vi "Nested Loops Solution.vi"() -> (3 "Solutions (Quantity)":i32[][](array[numeric]))   [LabVIEW 2018]
uses:
  ctl/Coin data--cluster.ctl
panel:
  out "No. solutions":i32
  out "Values (p)":i32[](array[numeric])
  out "Progress - current iteration values":i32[](array[numeric])
  out "Time taken (s)":dbl
  # "Beer money - Nested Loops/ Speedy solution"
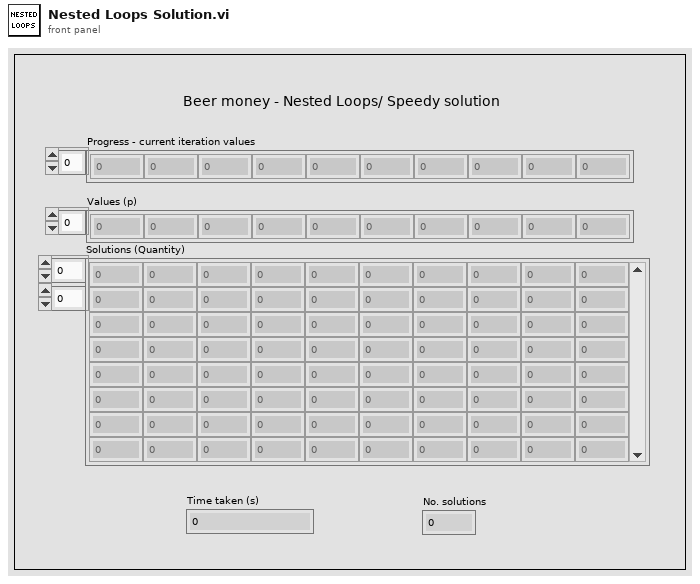
[diagram p1: front panel]
types:
  T1 = typedef "Coin data--cluster.ctl" = cluster{"Coin/note":i32, "Quantity":i32}
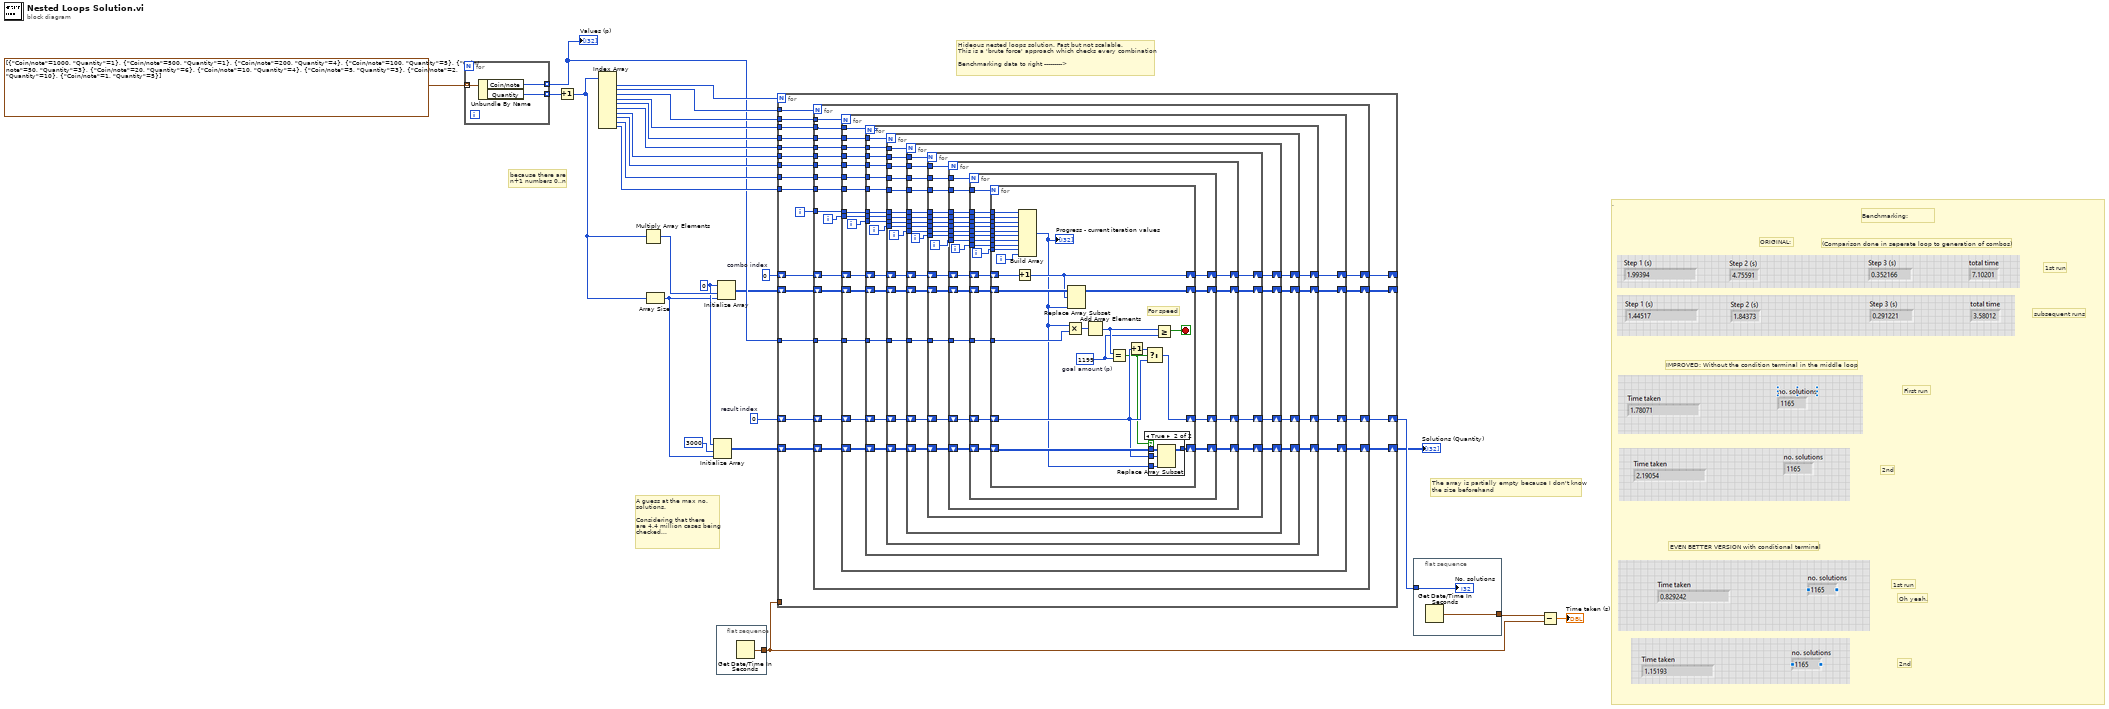
[diagram p0: block diagram]
diagram:
  w4 = 0 ("dimension size")
  w8 = 0  # result index
  w13 = 0  # combo index
  # "2nd"
  # "subsequent runs"
  # "The array is partially empty because I don't know\nthe size beforehand"
  # "Benchmarking:"
  # "(Comparison done in seperate loop to generation of combos)"
  # "1st run"
  # "Oh yeah."
  # "EVEN BETTER VERSION with conditional terminal"
  # "2nd"
  # "First run"
  # "IMPROVED: Without the condition terminal in the middle loop"
  # "A guess at the max no.\nsolutions.\n\nConsidering that there \nare 4.4 million cases being \nchecked..."
  # "ORIGINAL:"
  # "1st run"
  # "Hideous nested loops solution. Fast but not scalable.\nThis is a 'brute force' approach which checks every combination\n\nBenchmarking data to right --------->"
  # "because there are \nn+1 numbers 0..n"
  # "."
  n1 = for {
    tunnel: T1[] [{"Coin/note"=1000, "Quantity"=1}, {"Coin/note"=500, "Quantity"=1}, {"Coin/note"=200, "Quantity"=4}, {"Coin/note"=100, "Quantity"=5}, {"Coin/note"=50, "Quantity"=3}, {"Coin/note"=20, "Quantity"=6}, {"Coin/note"=10, "Quantity"=4}, {"Coin/note"=5, "Quantity"=3}, {"Coin/note"=2, "Quantity"=10}, {"Coin/note"=1, "Quantity"=5}] -> [w30] mode=indexing
    tunnel: [w29] -> w9 mode=indexing
    tunnel: [w28] -> w26 mode=indexing
    n2 = Unbundle By Name(w30) -> ("Coin/note"=w29:i32, "Quantity"=w28:i32)
  }
  "Values (p)" <- w9
  n3 = Increment(x=w26) -> (x+1=w12:i32[])
  n4 = Index Array(array=w12) -> (element #1=w24:i32, element #2=w23:i32, element #3=w22:i32, element #4=w21:i32, element #5=w20:i32, element #6=w19:i32, element #7=w18:i32, element #8=w17:i32, element #9=w16:i32, element #10=w15:i32)  [unwired: 10 in]
  n5 = Multiply Array Elements(1:w12) -> (0:w25:i32)
  n6 = Array Size(array=w12) -> (size(s)=w3:i32)
  n7 = Initialize Array(w4, 3000 ("dimension size"), w3) -> (w5:i32[][])
  n8 = flat-sequence {
    tunnel: [w31] -> w14
    frame #0 {
      n9 = Get Date/Time In Seconds() -> (seconds since 1Jan1904=w31:timestamp)
    }
  }
  n10 = Initialize Array(w4, w25, w3) -> (w7:i32[][])
  n11 = for {
    N: w24 -> [_]
    tunnel: w23 -> [w46]
    tunnel: w22 -> [w47]
    tunnel: w21 -> [w48]
    tunnel: w20 -> [w45]
    tunnel: w19 -> [w44]
    tunnel: w18 -> [w43]
    tunnel: w17 -> [w42]
    tunnel: w16 -> [w41]
    tunnel: w15 -> [w40]
    shift-right: [w50] -> _
    shift-left: w7 -> [w39]
    tunnel: w14 -> [_]
    shift-right: [w37] -> _
    shift-left: w13 -> [w38]
    tunnel: w9 -> [w36]
    shift-right: [w32] -> w6
    shift-left: w8 -> [w35]
    shift-right: [w33] -> w1
    shift-left: w5 -> [w34]
    i -> [w49]
    n12 = for {
      N: w46 -> [_]
      tunnel: w49 -> [w69]
      tunnel: w47 -> [w65]
      tunnel: w48 -> [w66]
      tunnel: w45 -> [w64]
      tunnel: w44 -> [w63]
      tunnel: w43 -> [w62]
      tunnel: w42 -> [w61]
      tunnel: w41 -> [w60]
      tunnel: w40 -> [w59]
      shift-right: [w68] -> w50
      shift-left: w39 -> [w58]
      shift-right: [w56] -> w37
      shift-left: w38 -> [w57]
      tunnel: w36 -> [w55]
      shift-right: [w51] -> w32
      shift-left: w35 -> [w54]
      shift-right: [w52] -> w33
      shift-left: w34 -> [w53]
      i -> [w67]
      n13 = for {
        N: w65 -> [_]
        tunnel: w69 -> [w88]
        tunnel: w67 -> [w87]
        tunnel: w66 -> [w84]
        tunnel: w64 -> [w83]
        tunnel: w63 -> [w82]
        tunnel: w62 -> [w81]
        tunnel: w61 -> [w80]
        tunnel: w60 -> [w79]
        tunnel: w59 -> [w78]
        shift-right: [w86] -> w68
        shift-left: w58 -> [w77]
        shift-right: [w75] -> w56
        shift-left: w57 -> [w76]
        tunnel: w55 -> [w74]
        shift-right: [w70] -> w51
        shift-left: w54 -> [w73]
        shift-right: [w71] -> w52
        shift-left: w53 -> [w72]
        i -> [w85]
        n14 = for {
          N: w84 -> [_]
          tunnel: w88 -> [w107]
          tunnel: w85 -> [w106]
          tunnel: w87 -> [w105]
          shift-right: [w104] -> w86
          shift-left: w77 -> [w103]
          tunnel: w83 -> [w102]
          tunnel: w82 -> [w101]
          tunnel: w81 -> [w100]
          tunnel: w80 -> [w99]
          tunnel: w79 -> [w98]
          tunnel: w78 -> [w97]
          shift-right: [w94] -> w75
          shift-left: w76 -> [w95]
          tunnel: w74 -> [w93]
          shift-right: [w89] -> w70
          shift-left: w73 -> [w92]
          shift-right: [w90] -> w71
          shift-left: w72 -> [w91]
          i -> [w96]
          n15 = for {
            N: w102 -> [_]
            tunnel: w107 -> [w126]
            tunnel: w106 -> [w125]
            tunnel: w105 -> [w124]
            shift-right: [w123] -> w104
            shift-left: w103 -> [w122]
            tunnel: w101 -> [w121]
            tunnel: w100 -> [w120]
            tunnel: w99 -> [w119]
            tunnel: w98 -> [w118]
            tunnel: w97 -> [w117]
            tunnel: w96 -> [w115]
            shift-right: [w113] -> w94
            shift-left: w95 -> [w114]
            tunnel: w93 -> [w112]
            shift-right: [w108] -> w89
            shift-left: w92 -> [w111]
            shift-right: [w109] -> w90
            shift-left: w91 -> [w110]
            i -> [w116]
            n16 = for {
              N: w121 -> [_]
              tunnel: w126 -> [w145]
              tunnel: w125 -> [w144]
              tunnel: w124 -> [w143]
              shift-right: [w142] -> w123
              shift-left: w122 -> [w141]
              tunnel: w120 -> [w140]
              tunnel: w119 -> [w139]
              tunnel: w118 -> [w138]
              tunnel: w117 -> [w137]
              tunnel: w116 -> [w136]
              tunnel: w115 -> [w134]
              shift-right: [w132] -> w113
              shift-left: w114 -> [w133]
              tunnel: w112 -> [w131]
              shift-right: [w127] -> w108
              shift-left: w111 -> [w130]
              shift-right: [w128] -> w109
              shift-left: w110 -> [w129]
              i -> [w135]
              n17 = for {
                N: w140 -> [_]
                tunnel: w145 -> [w164]
                tunnel: w144 -> [w163]
                tunnel: w143 -> [w162]
                shift-right: [w161] -> w142
                shift-left: w141 -> [w160]
                tunnel: w139 -> [w159]
                tunnel: w138 -> [w158]
                tunnel: w137 -> [w157]
                tunnel: w136 -> [w156]
                tunnel: w135 -> [w155]
                tunnel: w134 -> [w153]
                shift-right: [w151] -> w132
                shift-left: w133 -> [w152]
                tunnel: w131 -> [w150]
                shift-right: [w146] -> w127
                shift-left: w130 -> [w149]
                shift-right: [w147] -> w128
                shift-left: w129 -> [w148]
                i -> [w154]
                n18 = for {
                  N: w159 -> [_]
                  tunnel: w164 -> [w183]
                  tunnel: w163 -> [w182]
                  tunnel: w162 -> [w181]
                  shift-right: [w180] -> w161
                  shift-left: w160 -> [w179]
                  tunnel: w158 -> [w178]
                  tunnel: w157 -> [w177]
                  tunnel: w156 -> [w176]
                  tunnel: w155 -> [w175]
                  tunnel: w154 -> [w174]
                  tunnel: w153 -> [w172]
                  shift-right: [w170] -> w151
                  shift-left: w152 -> [w171]
                  tunnel: w150 -> [w169]
                  shift-right: [w165] -> w146
                  shift-left: w149 -> [w168]
                  shift-right: [w166] -> w147
                  shift-left: w148 -> [w167]
                  i -> [w173]
                  n19 = for {
                    N: w178 -> [_]
                    tunnel: w183 -> [w202]
                    tunnel: w182 -> [w201]
                    tunnel: w181 -> [w200]
                    shift-right: [w199] -> w180
                    shift-left: w179 -> [w198]
                    tunnel: w177 -> [w197]
                    tunnel: w176 -> [w196]
                    tunnel: w175 -> [w195]
                    tunnel: w174 -> [w194]
                    tunnel: w173 -> [w193]
                    tunnel: w172 -> [w191]
                    shift-right: [w189] -> w170
                    shift-left: w171 -> [w190]
                    tunnel: w169 -> [w188]
                    shift-right: [w184] -> w165
                    shift-left: w168 -> [w187]
                    shift-right: [w185] -> w166
                    shift-left: w167 -> [w186]
                    i -> [w192]
                    n20 = for {
                      N: w197 -> [_]
                      tunnel: w202 -> [w228]
                      tunnel: w201 -> [w227]
                      tunnel: w200 -> [w226]
                      shift-right: [w217] -> w199
                      shift-left: w198 -> [w218]
                      tunnel: w196 -> [w220]
                      tunnel: w195 -> [w219]
                      tunnel: w194 -> [w225]
                      tunnel: w193 -> [w224]
                      tunnel: w192 -> [w223]
                      tunnel: w191 -> [w221]
                      shift-right: [w215] -> w189
                      shift-left: w190 -> [w216]
                      tunnel: w188 -> [w213]
                      shift-right: [w211] -> w184
                      shift-left: w187 -> [w208]
                      shift-right: [w210] -> w185
                      shift-left: w186 -> [w209]
                      i -> [w222]
                      stop <- w205 stop-if-true
                      w206 = 1199  # goal amount (p)
                      # "For speed"
                      n21 = Increment(x=w216) -> (x+1=w215:i32)
                      n22 = Build Array(w228, w226, w227, w221, w220, w219, w225, w224, w223, w222) -> (w204:i32[])
                      "Progress - current iteration values" <- w204
                      n23 = Multiply(x=w204, y=w213) -> (x*y=w214:i32[])
                      n24 = Replace Array Subset(array=w218, new element=w204, index (row)=w215) -> (w217:i32[][])  [unwired: 1 in]
                      n25 = Add Array Elements(numeric array=w214) -> (sum=w207:i32)
                      n26 = Equal?(x=w207, y=w206) -> (x = y?=w203:bool)
                      n27 = Increment(x=w208) -> (x+1=w212:i32)
                      n28 = Select(t=w212, s=w203, f=w208) -> (s? t:f=w211:i32)
                      n29 = case shown="True" w203 {
                        tunnel: [w229 w233] -> w210
                        tunnel: w209 -> [w229 w232]
                        tunnel: w204 -> [_ w231]
                        tunnel: w208 -> [_ w230]
                        frame False {
                        }
                        frame True {
                          n30 = Replace Array Subset(array=w232, new element=w231, index (row)=w230) -> (w233:i32[][])  [unwired: 1 in]
                        }
                      }
                      n31 = Greater Or Equal?(x=w207, y=w206) -> (x >= y?=w205:bool)
                    }
                  }
                }
              }
            }
          }
        }
      }
    }
  }
  "Solutions (Quantity)" <- w1
  n32 = flat-sequence {
    tunnel: [w235] -> w11
    tunnel: w6 -> [w234]
    frame #0 {
      n33 = Get Date/Time In Seconds() -> (seconds since 1Jan1904=w235:timestamp)
      "No. solutions" <- w234
    }
  }
  n34 = Subtract(x=w11, y=w14) -> (x-y=→"Time taken (s)":dbl)
